vi "Increment_Number_Of_Experiments.vi"(10 "Experiments":T1(array[cluster]), 11 "Numeric":i32) -> (3 "f":i32)   [LabVIEW 2015]
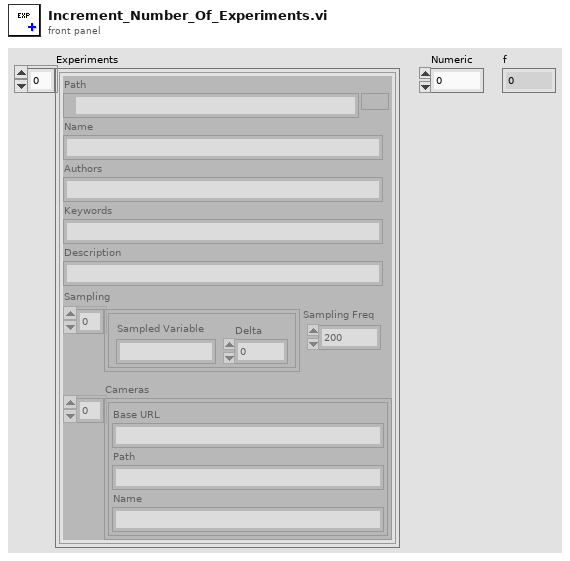
[diagram p1: front panel]
types:
  T1 = cluster{"Path":path, "Name":string, "Authors":string, "Keywords":string, "Description":string, "Cameras":cluster{"Base URL":string, "Path":string, "Name":string}[], "Sampling":cluster{"Sampled Variable":string, "Delta":dbl}[], "Sampling Freq":u32}[]
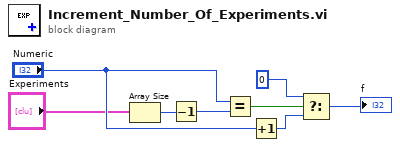
[diagram p0: block diagram]
diagram:
  n1 = Array Size(array="Experiments") -> (size(s)=w1:i32)
  n2 = Decrement(x=w1) -> (x-1=w8:i32)
  n3 = Equal?(x="Numeric", y=w8) -> (x = y?=w2:bool)
  n4 = Increment(x="Numeric") -> (x+1=w5:i32)
  n5 = Select(t=0 ("f"), s=w2, f=w5) -> (s? t:f=→"f":i32)
